vi "Register Process.vi"(6 "Forces Self to Run (F)":bool, 7 "Parent Call":T1, 8 "error in (no error)":errorcluster, 9 "Process Name (Optional)":string, 11 "SMO":refnum<class "SMO.lvclass">) -> (0 "error out":errorcluster, 3 "SMO out":refnum<class "SMO.lvclass">)   [LabVIEW 2013, in "SMO.lvclass"]
uses:
  SMO.lvclass
  Typedefs/Parent Call--Enum.ctl
panel:
  # "For instructions on how to use the JKI State Machine Objects, examples and video tutorials, visit:\nhttp://jki.net/state-machine-objects/\n\nJKI State Machine Objects™\nhttp://jki.net/state-machine-objects/\nCopyright (C) 2005-2015, JKI <info@jki.net>\nALL RIGHTS RESERVED"
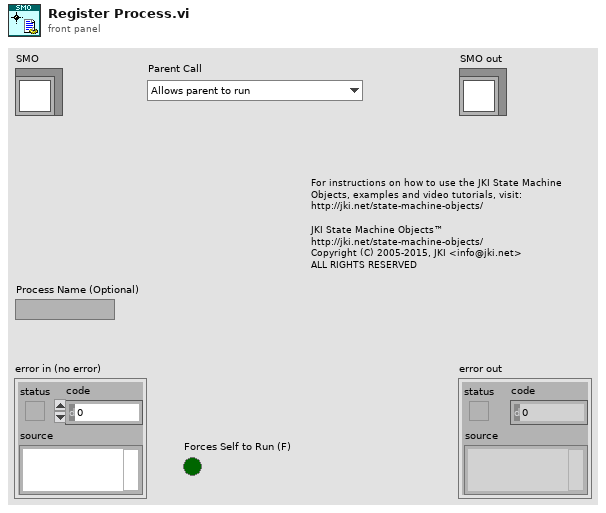
[diagram p1: front panel]
types:
  T1 = typedef "SMO.lvclass/Parent Call--Enum.ctl" = enum16{"Allows parent to run", "Does not request parent to run"}
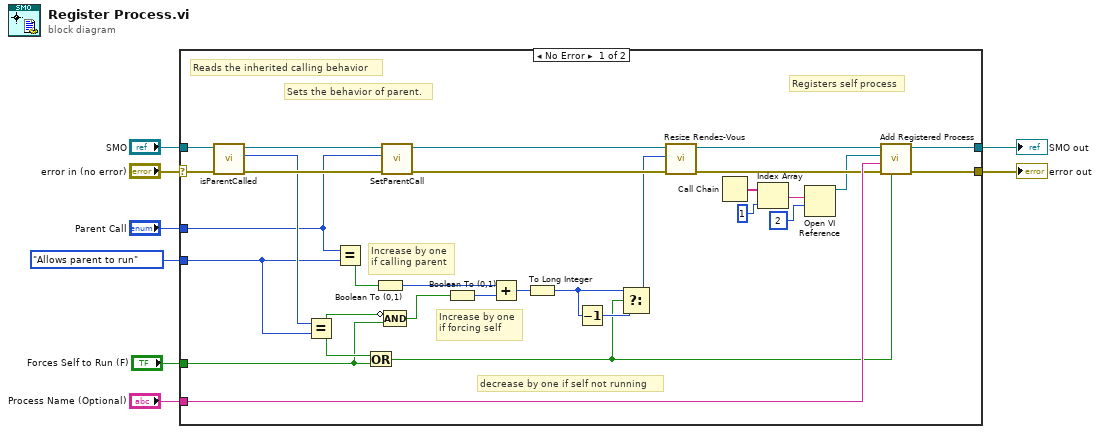
[diagram p0: block diagram]
diagram:
  n1 = case shown="No Error" "error in (no error)" {
    selector: "error in (no error)" -> [w24 w39]
    tunnel: "SMO" -> [w26 w40]
    tunnel: [w37 w40] -> w7
    tunnel: [w36 w39] -> w5
    tunnel: "Process Name (Optional)" -> [w38 _]
    tunnel: "Parent Call" -> [w21 _]
    tunnel: "Forces Self to Run (F)" -> [w17 _]
    tunnel: Parent_Call--Enum."Allows parent to run" ("y") -> [w20 _]
    frame No Error {
      # "Increase by one\nif forcing self"
      # "decrease by one if self not running"
      # "Registers self process"
      # "Sets the behavior of parent."
      # "Reads the inherited calling behavior"
      # "Increase by one\nif calling parent"
      n2 = call "isParentCalled.vi"("error in (no error)"=w24, "SMO in"=w26) -> ("error out"=w23:errorcluster, "Parent Call"=w22:T1, "SMO out"=w25:refnum<class "SMO.lvclass">)  [unwired: 7 in]
      n3 = Equal?(x=w22, y=w20) -> (x = y?=w18:bool)
      n4 = Equal?(x=w21, y=w20) -> (x = y?=w14:bool)
      n5 = Or(x=w18, y=w17) -> (x .or. y?=w10:bool)
      n6 = Boolean To (0,1)(Boolean=w14) -> (0, 1=w13:i16)
      n7 = call "SetParentCall.vi"("error in (no error)"=w23, "Parent Call"=w21, "SMO in"=w25) -> ("error out"=w27:errorcluster, "SMO out"=w28:refnum<class "SMO.lvclass">)  [unwired: 7 in]
      n8 = Compound Arithmetic op=AND(invert w18, w17) -> (w15:bool)
      n9 = Boolean To (0,1)(Boolean=w15) -> (0, 1=w12:i16)
      n10 = Add(x=w13, y=w12) -> (x+y=w11:i16)
      n11 = To Long Integer(number=w11) -> (32bit integer=w9:i32)
      n12 = Decrement(x=w9) -> (x-1=w16:i32)
      n13 = Select(t=w9, s=w10, f=w16) -> (s? t:f=w19:i32)
      n14 = call "Resize Rendez-Vous.vi"("error in (no error)"=w27, "Resize"=w19, "SMO"=w28) -> ("error out"=w35:errorcluster, "SMO out"=w34:refnum<class "SMO.lvclass">)  [unwired: 7 in]
      n15 = Call Chain() -> (call chain=w33:string[])
      n16 = Index Array(array=w33, index=1 ("Index")) -> (element=w31:string)
      n17 = Open VI Reference(vi path=w31, options=2) -> (vi reference=w29:refnum<vi>)  [unwired: 4 in, 1 out]
      n18 = call "Add Registered Process.vi"("Process Runs (T)"=w10, "error in (no error)"=w35, "Process Name (Optional)"=w38, "Process VI (Static VI Ref)"=w29, "SMO"=w34) -> ("error out"=w36:errorcluster, "SMO out"=w37:refnum<class "SMO.lvclass">)  [unwired: 5 in]
    }
    frame Error {
    }
  }
  "error out" <- w5
  "SMO out" <- w7
